vi "CoMP-S TDMS Create.vi"(8 "error in (no error)":errorcluster, 10 "Prefix":string, 11 "Default Folder Path":string="C:\\SCMP Logs\\CoMP-S Mechanism TDMS\\") -> (0 "error out":errorcluster, 2 "file name":string, 3 "tdms file out":refnum<k34>, 5 "date/time string":string)   [LabVIEW 2014]
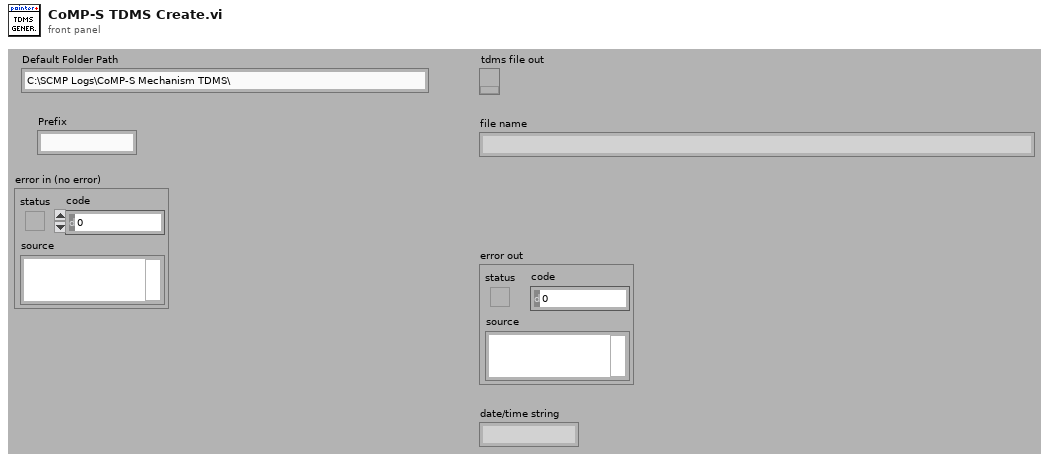
[diagram p1: front panel]
types:
  T1 = enum16{"open", "open or create", "create or replace", "create", "open (read-only)"}
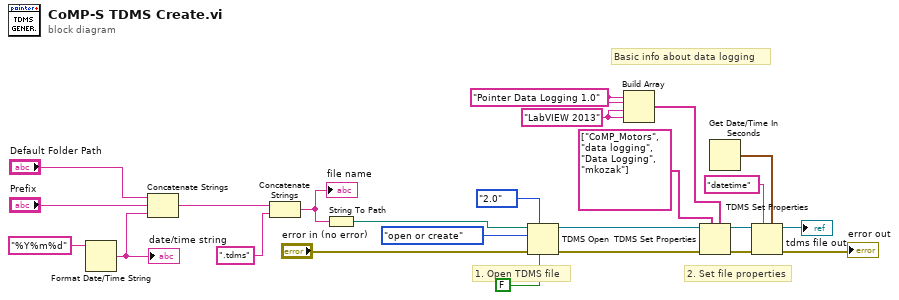
[diagram p0: block diagram]
diagram:
  w19 = "LabVIEW 2013" ("title")
  w20 = "Pointer Data Logging 1.0" ("name")
  # "2. Set file properties"
  # "1. Open TDMS file"
  # "Basic info about data logging"
  n1 = Format Date/Time String(time format string (%c)="%Y%m%d") -> (date/time string=w23:string)  [unwired: 2 in]
  "date/time string" <- w23
  n2 = Concatenate Strings("Default Folder Path", "Prefix", w23) -> (w24:string)
  n3 = Concatenate Strings(w24, ".tdms") -> (w5:string)
  "file name" <- w5
  n4 = String To Path(string=w5) -> (path=w6:path)
  n5 = TDMS Open(6:FALSE ("disable buffering (T)"), 7:enum16{"1.0", "2.0"}."2.0" ("file format version (2.0)"), 8:"error in (no error)", 10:T1."open or create" ("operation"), 11:w6) -> (0:w11:errorcluster, 3:w12:refnum<k34>)  [unwired: 2 in]
  n6 = Build Array(w20, w20, w19, w19) -> (w18:string[])
  n7 = TDMS Set Properties(5:w18, 7:string[] ["CoMP_Motors", "data logging", "Data Logging", "mkozak"] ("property names"), 8:w11, 11:w12) -> (0:w17:errorcluster, 3:w16:refnum<k34>)  [unwired: 4 out]
  n8 = Get Date/Time In Seconds() -> (seconds since 1Jan1904=w14:timestamp)
  n9 = TDMS Set Properties(5:w14, 7:"datetime", 8:w17, 11:w16) -> (0:→"error out":errorcluster, 3:→"tdms file out":refnum<k34>)  [unwired: 4 out]
